vi "zmq init.vi"(8 "error in (no error)":errorcluster, 11 "io_threads_":i32) -> (0 "error out":errorcluster, 3 "function return":u32)   [LabVIEW 2025, in "LibZMQ.lvlib"]
doc: "ZMQ_EXPORT void *zmq_init (int io_threads_);"
uses:
  LibZMQ.lvlib
  LV/LibZMQ/libzmq/lv_x86/bin/Release/libzmq-v143-mt-4_3_6.dll
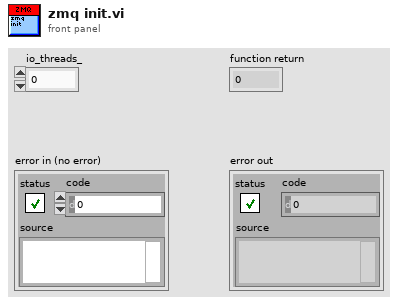
[diagram p1: front panel]
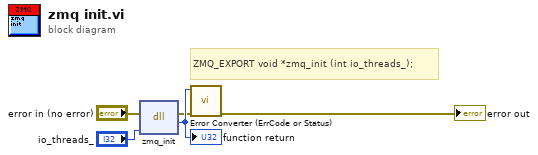
[diagram p0: block diagram]
diagram:
  # "ZMQ_EXPORT void *zmq_init (int io_threads_);"
  n1 = dll-call lib="C:/LV/LibZMQ/libzmq/lv_x86/bin/Release/libzmq-v143-mt-4_3_6.*" fn="zmq_init"(error in="error in (no error)", "io_threads_"="io_threads_") -> (error out=w2:errorcluster, w5:u32)  [unwired: 3 in, 1 out]
  "function return" <- w5
  n2 = call "Error Converter (ErrCode or Status).vi"("error in (no error)"=w2, "error code"=w5) -> ("error out"=→"error out":errorcluster)  [unwired: 9 in]
